vi "CAN Filter Init.vi"(9 "pFilterConfig":T1, 10 "CANIndex":u8, 11 "DevHandle":i32) -> (1 "pFilterConfig out":T1, 3 "function return":i32)   [LabVIEW 2010, in "usb2can.lvlib"]
doc: "int WINAPI CAN_Filter_Init(int DevHandle, unsigned char CANIndex, CAN_FILTER_CONFIG *pFilterConfig);"
uses:
  usb2can.lvlib
  USB2XXX.dll
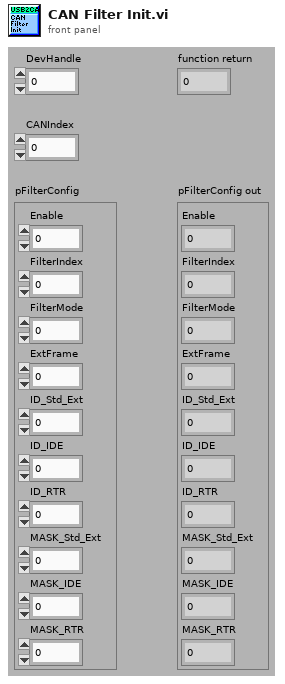
[diagram p1: front panel]
types:
  T1 = cluster{"Enable":u8, "FilterIndex":u8, "FilterMode":u8, "ExtFrame":u8, "ID_Std_Ext":u32, "ID_IDE":u32, "ID_RTR":u32, "MASK_Std_Ext":u32, "MASK_IDE":u32, "MASK_RTR":u32}
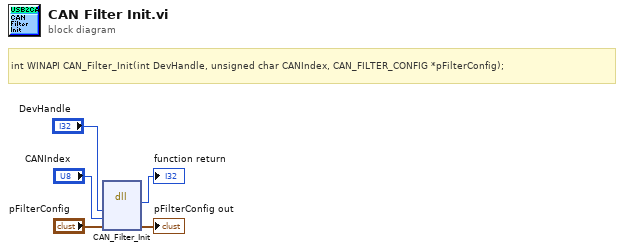
[diagram p0: block diagram]
diagram:
  # "int WINAPI CAN_Filter_Init(int DevHandle, unsigned char CANIndex, CAN_FILTER_CONFIG *pFilterConfig);"
  n1 = dll-call lib="E:/Projects/USB2XXX_Example/sdk/api/Labview/usb2can/USB2XXX.*" fn="CAN_Filter_Init"("DevHandle"="DevHandle", "CANIndex"="CANIndex", "pFilterConfig"="pFilterConfig") -> (→"function return":i32, "pFilterConfig"=→"pFilterConfig out":T1)  [unwired: 5 in, 2 out]
